vi "Chroma 1905x Series 488.2 Cmd -RST.vi"(8 "error in (no error)":errorcluster, 11 "VISA resource name":refnum<visa-resource-name>) -> (0 "error out":errorcluster, 3 "VISA resource name out":refnum<visa-resource-name>)   [LabVIEW 2025]
panel:
  # "*RST"
  # "Reset Device"
  # "NOTE: After command there is a 4 sec delay"
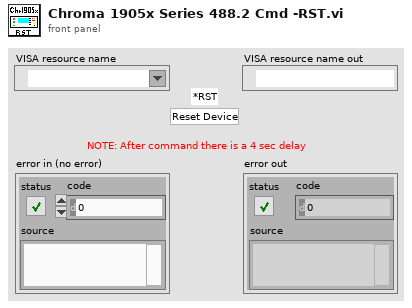
[diagram p1: front panel]
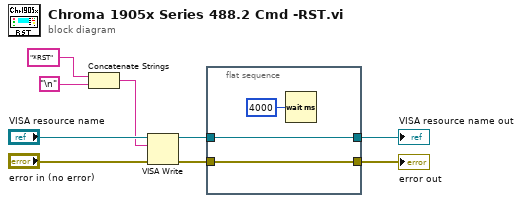
[diagram p0: block diagram]
diagram:
  n1 = Concatenate Strings("*RST", "\n") -> (w1:string)
  n2 = VISA Write(VISA resource name="VISA resource name", write buffer=w1, error in (no error)="error in (no error)") -> (VISA resource name out=w4:refnum<visa-resource-name>, error out=w6:errorcluster)  [unwired: 1 out]
  n3 = flat-sequence {
    tunnel: w6 -> [w12]
    tunnel: [w12] -> w5
    tunnel: w4 -> [w11]
    tunnel: [w11] -> w2
    frame #0 {
      n4 = Wait (ms)(milliseconds to wait=u32 4000) -> ()  [unwired: 1 out]
    }
  }
  "error out" <- w5
  "VISA resource name out" <- w2
